vi "resetEvent.vi"(8 "error in (no error)":errorcluster, 11 "ActionEditor in":refnum<class "ActionEditor.lvclass">) -> (0 "error out":errorcluster, 3 "ActionEditor out":refnum<class "ActionEditor.lvclass">)   [LabVIEW 2011, in "Views.lvlib" / "ScriptEditor.lvlib" / "ActionEditor.lvclass"]
uses:
  ActionEditor.lvclass
  Tools/Scripting/ScriptingEvent/ScriptEvent.lvclass
  ActionEditor.lvclass/ActionEditor.ctl
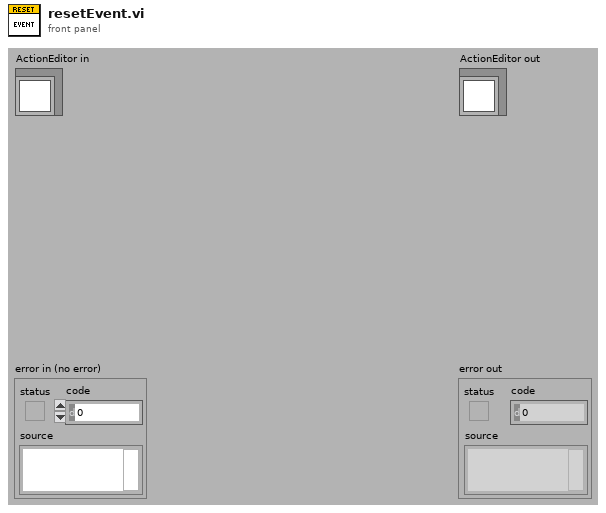
[diagram p1: front panel]
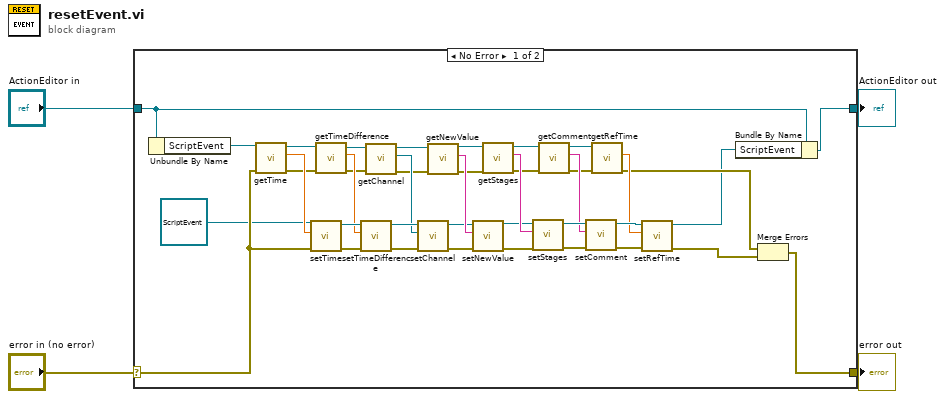
[diagram p0: block diagram]
diagram:
  n1 = case shown="No Error" "error in (no error)" {
    selector: "error in (no error)" -> [w40 w46]
    tunnel: [w16 w46] -> w3
    tunnel: [w13 w45] -> w1
    tunnel: "ActionEditor in" -> [w14 w45]
    frame No Error {
      n2 = Unbundle By Name(w14) -> ("ScriptEvent"=w44:refnum<class "ScriptEvent.lvclass">)
      n3 = call "getTime.vi"("error in (no error)"=w40, "ScriptEvent.lvclass in"=w44) -> ("error out"=w41:errorcluster, "time"=w43:dbl, "ScriptEvent.lvclass out"=w42:refnum<class "ScriptEvent.lvclass">)  [unwired: 7 in]
      n4 = call "setTime.vi"("error in (no error)"=w40, "time"=w43, "ScriptEvent.lvclass in"=refnum<class "ScriptEvent.lvclass"> refnum ("Tools.lvlib:Scripting.lvlib:ScriptEvent.lvclass")) -> ("error out"=w38:errorcluster, "ScriptEvent.lvclass out"=w39:refnum<class "ScriptEvent.lvclass">)  [unwired: 7 in]
      n5 = call "getTimeDifference.vi"("error in (no error)"=w41, "ScriptEvent.lvclass in"=w42) -> ("error out"=w36:errorcluster, "time difference"=w37:dbl, "ScriptEvent.lvclass out"=w35:refnum<class "ScriptEvent.lvclass">)  [unwired: 7 in]
      n6 = call "setTimeDifference.vi"("error in (no error)"=w38, "time difference"=w37, "ScriptEvent.lvclass in"=w39) -> ("error out"=w32:errorcluster, "ScriptEvent.lvclass out"=w34:refnum<class "ScriptEvent.lvclass">)  [unwired: 7 in]
      n7 = call-dynamic "getChannel.vi"("error in (no error)"=w36, "ScriptEvent.lvclass in"=w35) -> ("error out"=w30:errorcluster, "Channel.lvclass"=w33:refnum<class "Channel.lvclass">, "ScriptEvent.lvclass out"=w31:refnum<class "ScriptEvent.lvclass">)  [unwired: 7 in]
      n8 = call-dynamic "setChannel.vi"("error in (no error)"=w32, "Channel.lvclass"=w33, "ScriptEvent.lvclass in"=w34) -> ("error out"=w27:errorcluster, "ScriptEvent.lvclass out"=w28:refnum<class "ScriptEvent.lvclass">)  [unwired: 7 in]
      n9 = call "getNewValue.vi"("error in (no error)"=w30, "ScriptEvent.lvclass in"=w31) -> ("error out"=w25:errorcluster, "newValue"=w29:string, "ScriptEvent.lvclass out"=w26:refnum<class "ScriptEvent.lvclass">)  [unwired: 7 in]
      n10 = call "setNewValue.vi"("error in (no error)"=w27, "newValue"=w29, "ScriptEvent.lvclass in"=w28) -> ("error out"=w22:errorcluster, "ScriptEvent.lvclass out"=w23:refnum<class "ScriptEvent.lvclass">)  [unwired: 7 in]
      n11 = call "getStages.vi"("error in (no error)"=w25, "ScriptEvent.lvclass in"=w26) -> ("error out"=w20:errorcluster, "Stage"=w24:string, "ScriptEvent.lvclass out"=w21:refnum<class "ScriptEvent.lvclass">)  [unwired: 7 in]
      n12 = call-dynamic "setStages.vi"("error in (no error)"=w22, "Stage"=w24, "ScriptEvent.lvclass in"=w23) -> ("error out"=w18:errorcluster, "ScriptEvent.lvclass out"=w19:refnum<class "ScriptEvent.lvclass">)  [unwired: 7 in]
      n13 = call "getComment.vi"("error in (no error)"=w20, "ScriptEvent.lvclass in"=w21) -> ("error out"=w12:errorcluster, "comment"=w17:string, "ScriptEvent.lvclass out"=w11:refnum<class "ScriptEvent.lvclass">)  [unwired: 7 in]
      n14 = call-dynamic "setComment.vi"("error in (no error)"=w18, "comment"=w17, "ScriptEvent.lvclass in"=w19) -> ("error out"=w9:errorcluster, "ScriptEvent.lvclass out"=w10:refnum<class "ScriptEvent.lvclass">)  [unwired: 7 in]
      n15 = call "getRefTime.vi"("error in (no error)"=w12, "ScriptEvent.lvclass in"=w11) -> ("error out"=w7:errorcluster, "refTime"=w8:dbl)  [unwired: 7 in, 1 out]
      n16 = call "setRefTime.vi"("error in (no error)"=w9, "refTime"=w8, "ScriptEvent.lvclass in"=w10) -> ("error out"=w6:errorcluster, "ScriptEvent.lvclass out"=w5:refnum<class "ScriptEvent.lvclass">)  [unwired: 7 in]
      n17 = Bundle By Name(cluster=w14, "ScriptEvent"=w5) -> (w13:refnum<class "ActionEditor.lvclass">)
      n18 = Merge Errors(w7, w6) -> (w16:errorcluster)
    }
    frame Error {
    }
  }
  "error out" <- w3
  "ActionEditor out" <- w1
